vi "CheckPaths.vi"(9 "Output Path":path, 10 "New VI Path":path, 11 "Old VI Path":path) -> (0 "error out":errorcluster, 1 "Output Path Out":path, 2 "New VI Path Out":path, 3 "Old VI Path Out":path)   [LabVIEW 2017]
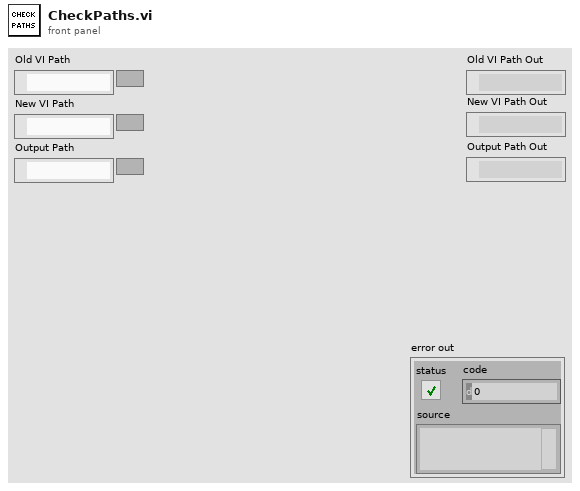
[diagram p1: front panel]
types:
  T1 = cluster{"Path":path, "Option Name":string, "Must Exist?":bool}
  T2 = cluster{"Path":path, "Option Name":string, "Must Exist?":bool}[]
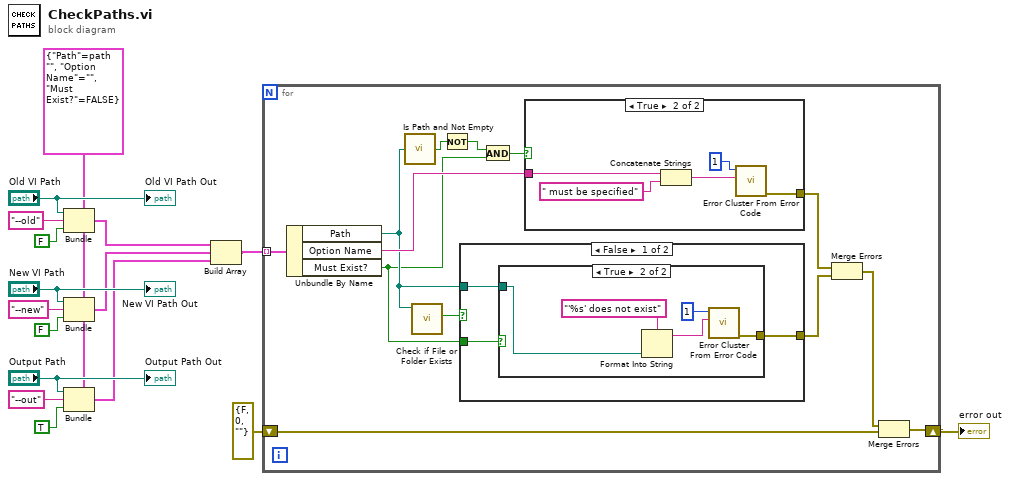
[diagram p0: block diagram]
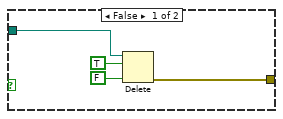
[diagram p2: hidden frame]
diagram:
  w3 = T1 {"Path"=path "", "Option Name"="", "Must Exist?"=FALSE} ("output cluster")
  n1 = Bundle(cluster=w3, "Path"="Old VI Path", "Option Name"="--old", "Must Exist?"=FALSE) -> (w12:T1)
  n2 = Bundle(cluster=w3, "Path"="New VI Path", "Option Name"="--new", "Must Exist?"=FALSE) -> (w11:T1)
  n3 = Bundle(cluster=w3, "Path"="Output Path", "Option Name"="--out", "Must Exist?"=TRUE) -> (w8:T1)
  n4 = Build Array(w12, w11, w8) -> (w7:T2)
  n5 = for {
    tunnel: w7 -> [w29] mode=indexing
    shift-right: [w21] -> w1
    shift-left: errorcluster {"status"=FALSE, "code"=0, "source"=""} ("error IO") -> [w23]
    n6 = Unbundle By Name(w29) -> ("Path"=w26:path, "Option Name"=w28:string, "Must Exist?"=w20:bool)
    n7 = call <vilib>:"Is Path and Not Empty.vi"("path"=w26) -> ("Is Path and Not Empty?"=w17:bool)  [unwired: 4 in]
    n8 = call <vilib>:"Check if File or Folder Exists.vi"("path"=w26) -> ("file or folder exists?"=w27:bool)  [unwired: 8 in, 2 out]
    n9 = Not(x=w17) -> (.not. x?=w18:bool)
    n10 = case shown="False" w27 {
      tunnel: [w32 _] -> w24
      tunnel: w20 -> [w31 _]
      tunnel: w26 -> [w30 _]
      frame False {
        n11 = case shown="True" w31 {
          tunnel: [w33 w41] -> w32
          tunnel: w30 -> [w34 w37]
          frame False {
            n12 = Delete(path (use dialog)=w34, entire hierarchy (F)=TRUE, confirm (F)=FALSE) -> (error out=w33:errorcluster)  [unwired: 2 in, 2 out]
          }
          frame True {
            n13 = Format Into String(format string="'%s' does not exist", w37) -> (resulting string=w39:string)  [unwired: 2 in, 1 out]
            n14 = call <vilib>:"Error Cluster From Error Code.vi"("error message (\"\")"=w39, "error code (0)"=1) -> ("error out"=w41:errorcluster)  [unwired: 7 in]
          }
        }
      }
      frame True {
      }
    }
    n15 = And(x=w18, y=w20) -> (x .and. y?=w19:bool)
    n16 = case shown="True" w19 {
      tunnel: w28 -> [_ w46]
      tunnel: [_ w42] -> w25
      frame False {
      }
      frame True {
        n17 = Concatenate Strings(w46, " must be specified" ("error message (\"\")")) -> (w44:string)
        n18 = call <vilib>:"Error Cluster From Error Code.vi"("error message (\"\")"=w44, "error code (0)"=1) -> ("error out"=w42:errorcluster)  [unwired: 7 in]
      }
    }
    n19 = Merge Errors(w25, w24) -> (w22:errorcluster)
    n20 = Merge Errors(w22, w23) -> (w21:errorcluster)
  }
  "error out" <- w1
  "Old VI Path Out" <- "Old VI Path"
  "New VI Path Out" <- "New VI Path"
  "Output Path Out" <- "Output Path"
